vi "Define Test Suite (Report).vi"(8 "error in (no error)":errorcluster, 9 "Test Report":refnum<class "Test Report.lvclass">, 10 "Interactive":bool, 11 "Label (VI Title)":string) -> (0 "error out":errorcluster, 3 "Test Suite":refnum<class "Test Suite.lvclass">)   [LabVIEW 2009, in "Caraya.lvlib" / "Test Suite.lvclass"]
doc: "Registers the calling VI as a test suite. If Interactive is True, the interactive user interface is opened when the test suite is executed. If the Report Path is set, a report file will be generated with the test results.\n\n--\nCopyright © 2015 JKI All rights reserved.\n\nAuthor: Tomi Maila <tomi.maila@jki.net>\n\nThis library is provided \"AS IS\" ,WITHOUT WARRANTIES OR\nCONDITIONS OF ANY KIND, either express or implied.\n\nJKI -- jki.net"
uses:
  Test Suite.lvclass
  Test Report/Test Report.lvclass
  Test Assert Factory/Test Assert Factory.lvclass
  Assert Factory/Assert Factory.lvclass
  Test Suite.lvclass/Test Suite.ctl
  Test Manager/Test Manager.lvclass
  Caraya.lvlib
  Assert Factory Manager/Assert Factory Manager.lvclass
panel:
  # "Copyright © 2015 JKI All rights reserved.\n\nAuthor: Tomi Maila <tomi.maila@jki.net>\n\nThis library is provided \"AS IS\" ,WITHOUT WARRANTIES OR\nCONDITIONS OF ANY KIND, either express or implied.\n\nJKI -- jki.net"
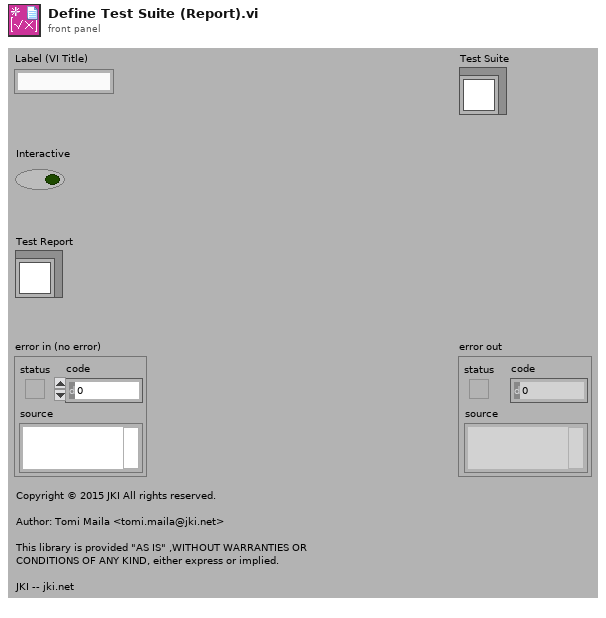
[diagram p1: front panel]
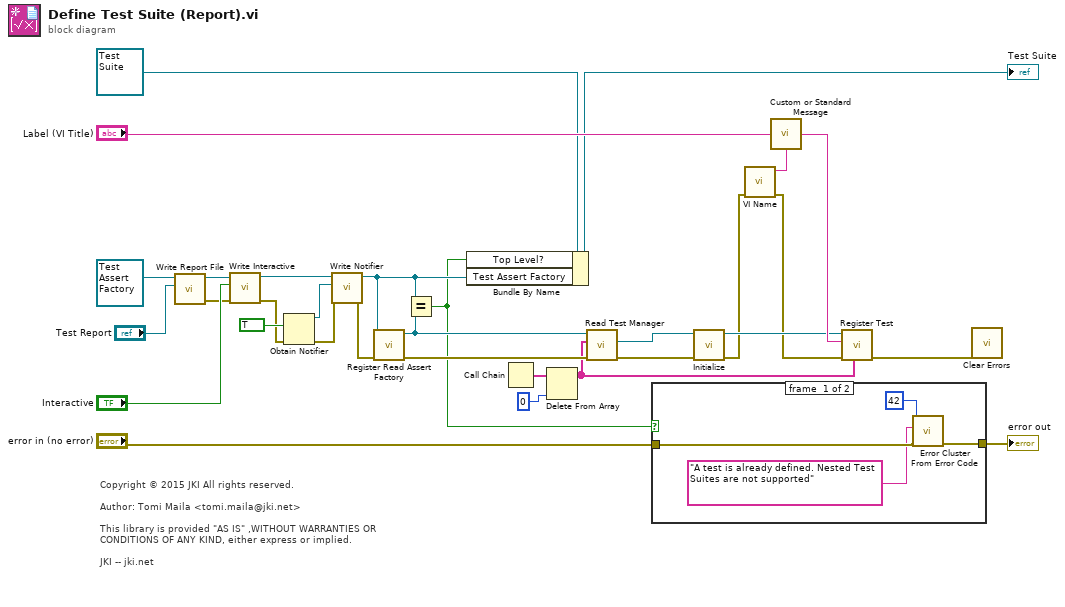
[diagram p0: block diagram]
diagram:
  # "Copyright © 2015 JKI All rights reserved.\n\nAuthor: Tomi Maila <tomi.maila@jki.net>\n\nThis library is provided \"AS IS\" ,WITHOUT WARRANTIES OR\nCONDITIONS OF ANY KIND, either express or implied.\n\nJKI -- jki.net"
  n1 = call "Write Report File.vi"("Test Report"="Test Report", "Test Assert Factory in"=refnum<class "Test Assert Factory.lvclass"> refnum ("Caraya.lvlib:Test Assert Factory.lvclass")) -> ("error out"=w26:errorcluster, "Test Assert Factory out"=w28:refnum<class "Test Assert Factory.lvclass">)  [unwired: 8 in]
  n2 = call "Write Interactive.vi"("error in (no error)"=w26, "Interactive"="Interactive", "Test Assert Factory in"=w28) -> ("error out"=w20:errorcluster, "Test Assert Factory out"=w23:refnum<class "Test Assert Factory.lvclass">)  [unwired: 7 in]
  n3 = Obtain Notifier(notification data type=TRUE, error in (no error)=w20) -> (notifier out=w18:refnum<notifier>, error out=w19:errorcluster)  [unwired: 2 in, 1 out]
  n4 = call "Write Notifier.vi"("error in (no error)"=w19, "notifier"=w18, "Test Assert Factory in"=w23) -> ("error out"=w24:errorcluster, "Test Assert Factory out"=w7:refnum<class "Test Assert Factory.lvclass">)  [unwired: 7 in]
  n5 = call "Register Read Assert Factory.vi"("error in (no error)"=w24, "Assert Factory"=w7) -> ("error out"=w30:errorcluster, "Assert Factory"=w6:refnum<class "Assert Factory.lvclass">)  [unwired: 8 in]
  n6 = Equal?(x=w7, y=w6) -> (x = y?=w3:bool)
  n7 = Bundle By Name(cluster=refnum<class "Test Suite.lvclass"> refnum ("Test Suite"), "Top Level?"=w3, "Test Assert Factory"=w7) -> (→"Test Suite":refnum<class "Test Suite.lvclass">)
  n8 = Call Chain() -> (call chain=w9:string[])
  n9 = Delete From Array(array=w9, index=0) -> (array with subset deleted=w8:string[])  [unwired: 1 in, 1 out]
  n10 = call-dynamic "Read Test Manager.vi"("error in (no error)"=w30, "VI Call Chain"=w8, "Assert Factory in"=w6) -> ("error out"=w14:errorcluster, "Test Manager"=w2:refnum<class "Test Manager.lvclass">)  [unwired: 6 in, 1 out]
  n11 = case shown="False" w3 {
    tunnel: [w35 w36] -> w5
    tunnel: "error in (no error)" -> [w34 w36]
    frame #0 {
      n12 = call <vilib>:"Error Cluster From Error Code.vi"("error in (no error)"=w34, "error message (\"\")"="A test is already defined. Nested Test Suites are not supported" ("error message (\"\")"), "error code (0)"=42) -> ("error out"=w35:errorcluster)  [unwired: 6 in]
    }
    frame #1 {
    }
  }
  "error out" <- w5
  n13 = call-dynamic "Initialize.vi"("error in (no error)"=w14, "Test Manager in"=w2) -> ("error out"=w13:errorcluster, "Test Manager out"=w15:refnum<class "Test Manager.lvclass">)  [unwired: 8 in]
  n14 = call "VI Name.vi"("error in (no error)"=w13) -> ("error out"=w12:errorcluster, "VI Name"=w17:string)  [unwired: 9 in]
  n15 = call "Custom or Standard Message.vi"("Custom Message"="Label (VI Title)", "Standard Message"=w17) -> ("Message"=w16:string)
  n16 = call-dynamic "Register Test.vi"("Call Chain"=w8, "error in (no error)"=w12, "Name"=w16, "Test Manager in"=w15) -> ("error out"=w11:errorcluster)  [unwired: 6 in, 1 out]
  n17 = call <vilib>:"Clear Errors.vi"("error in (no error)"=w11) -> ()  [unwired: 6 in, 1 out]
